vi "MagnetTop.vi"(8 "Queue to UI":T10, 11 "Module queue":T10) -> ()   [LabVIEW 2022 SP3, in "Magnet module.lvlib"]
doc: "Magnet module controls: power supply unit (PSU/SMS) and temperature monitor (TM/LSC218).\nPSU controls mainly: switch heater and ramping of current which runs throught coil.\nTM controls temperature of switch, coil and cryostat.\nMessage for magnet is a cluster that contains: {(enum) Command , (variant) Data}\nFor simplifieing of documentation, the Command is noted as a name of instruction, and Data is represented by a requered datatype (mostly cluster) name.\nCommands:\nInitialize(Magnet Config Constants) - Sugesstion: Load configuration constants from configuration file.\nSet field (Set field{B, R, cr}) - B-field[T], R-ramp[A/s], cr - custom ramp[bool].\nSwitch mode(mode) - to persistant, or to ramping.\nBlackout() - undone functionality of emergency deenergizing.\nUpdate() - Important! This triggers update of data from instruments. Shoud occure in regular intervals as priority message.\nResponses:\nMagnet initialized ();\nTM revision(temperature monitor revision);\nMagnet init error(error);\nSetting field(Set Field{B, R, cr});\nWarning(string);\nSwitching to(mode);\nUpdate error(error);\nTM update(TM sensors);\nPSU update(PSU data);\nMagnet status();"
uses:
  Magnet module.lvlib
  Messenger service/Data types/Mailbox address.ctl
  <instrlib>/SMS 120/Public/PSU Status.ctl
  ctl/Cryostat temperature sensors.ctl
  ctl/Overall status.ctl
  ctl/SetField data.ctl
  ctl/Magnet mode public.ctl
  ctl/Actual magnet state.ctl
  ctl/Magnet mode.ctl
  ctl/RampingOutput.ctl
  ctl/Magnet config constants.ctl
  Messenger service/Data types/Module name.ctl
  ctl/Magnet Orders.ctl
  ctl/MSG to magnet.ctl
  <instrlib>/SMS 120/Cryogenic Ltd SMSXXX.lvlib
  Messenger service/MessengerLib.lvlib
panel:
  out "Ended":bool=TRUE
  out "Magnet Constants":T1={"Switch resistant [K]"=5.0, "Switch superconducting [K]"=4.0, "First stage critical temperature [K]"=50.0, "Second stage critical temperature [K]"=5.0, "Inner magnet critical temperature [K]"=6.0, "Outer magnet critical temperature [K]"=5.0, "Field Constant [T/A]"=0.14911, "Maximum Current [A]"=107.3, "Maximum field [T]"=16.0, "Maximum source ramp [A/s]"=0.5, "Source precision [T]"=2e-05, "Ramp limits [A/s]"=[0.0506, 0.038, 0.0285, 0.0213, 0.0104], "Field limits [T]"=[3.0, 9.6, 13.3, 15.5, 16.0], "SMS"="", "LSC218"=""}
  out "Overall status":T2={"Desired"={"Field [T]"=0.0, "Ramp [T/s]"=0.0, "Custom Ramp?"=TRUE, "Mode"=enum."Persistant"}, "Actual"={"Mode"=enum."Persistant", "Ramping output"=enum."At Target", "Ready for change"=FALSE, "Switch heater"=FALSE, "Cooler Overheat"=FALSE, "Coil overheat"=FALSE, "Energized"=FALSE, "Output [T]"=0.0, "Field [T]"=0.0, "Ramp[T/s]"=0.0, "Switch\ntemperature [K]"=1.0, "Voltage [V]"=0.0, "Current direction"=FALSE}}
  out "Temperatures":T8[](array[typedef]) {"Time stamp" format="%<%H:%M:%S%2u\n%Y/%m/%d>T"}
  out "PSU Status Out":T9 {"Trip Current" format="%.3f"; "Trip Field" format="%.4f"; "Voltage" format="%.2f"; "Field Constant" format="%.6f"; "MID Setpoint (T)" format="%.4f"; "MID Setpoint (A)" format="%.3f"; "MAX Setpoint (T)" format="%.4f"; "MAX Setpoint (A)" format="%.3f"; "Heater Voltage" format="%.2f"; "V Limit (V)" format="%.2f"; "Ramp Rate (A/s)" format="%.3f"; "Output (A)" format="%.3f"; "Output (T)" format="%.4f"; "Persistent Current" format="%.3f"; "Persistent Field" format="%.4f"}
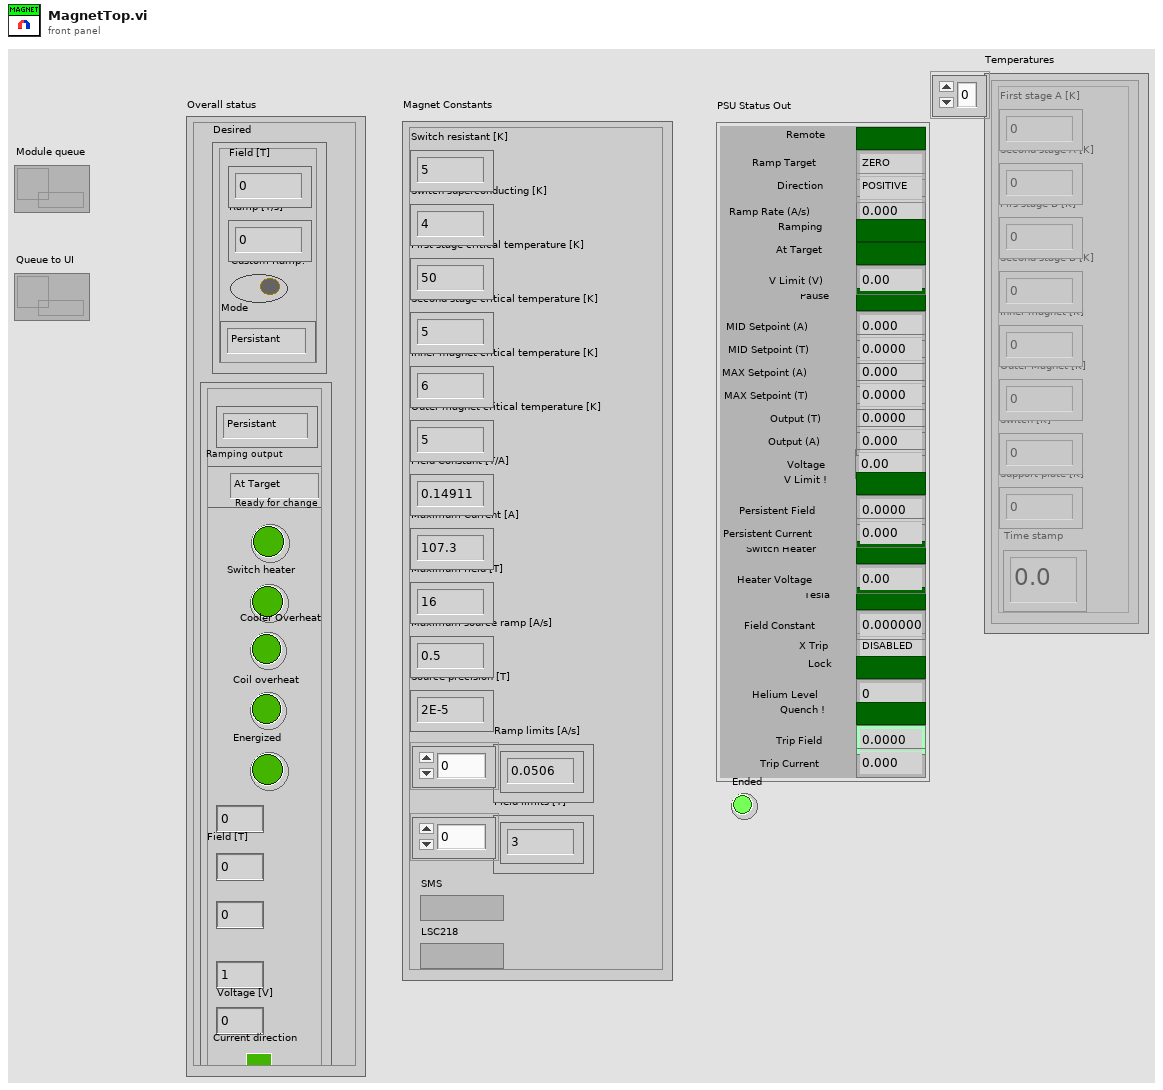
[diagram p1: front panel]
types:
  T1 = typedef "Magnet module.lvlib/Magnet config constants.ctl" = cluster{"Switch resistant [K]":dbl, "Switch superconducting [K]":dbl, "First stage critical temperature [K]":dbl, "Second stage critical temperature [K]":dbl, "Inner magnet critical temperature [K]":dbl, "Outer magnet critical temperature [K]":dbl, "Field Constant [T/A]":dbl, "Maximum Current [A]":dbl, "Maximum field [T]":dbl, "Maximum source ramp [A/s]":dbl, "Source precision [T]":dbl, "Ramp limits [A/s]":dbl[], "Field limits [T]":dbl[], "SMS":refnum<visa-resource-name>, "LSC218":refnum<visa-resource-name>}
  T2 = typedef "Magnet module.lvlib/Overall status.ctl" = cluster{"Desired":T3, "Actual":T5}
  T3 = typedef "Magnet module.lvlib/SetField data.ctl" = cluster{"Field [T]":dbl, "Ramp [T/s]":dbl, "Custom Ramp?":bool, "Mode":T4}
  T4 = typedef "Magnet module.lvlib/Magnet mode public.ctl" = enum16{"Persistant", "Ramping"}
  T5 = typedef "Magnet module.lvlib/Actual magnet state.ctl" = cluster{"Mode":T6, "Ramping output":T7, "Ready for change":bool, "Switch heater":bool, "Cooler Overheat":bool, "Coil overheat":bool, "Energized":bool, "Output [T]":dbl, "Field [T]":dbl, "Ramp[T/s]":dbl, "Switch\ntemperature [K]":dbl, "Voltage [V]":dbl, "Current direction":bool}
  T6 = typedef "Magnet module.lvlib/Magnet mode.ctl" = enum16{"Persistant", "Switching", "Ramping", "Quenched"}
  T7 = typedef "Magnet module.lvlib/RampingOutput.ctl" = enum16{"At Target", "Go up", "Go down"}
  T8 = typedef "Magnet module.lvlib/Cryostat temperature sensors.ctl" = cluster{"First stage A [K]":dbl, "Second stage A [K]":dbl, "Firs stage B [K]":dbl, "Second stage B [K]":dbl, "Inner magnet [K]":dbl, "Outer Magnet [K]":dbl, "Switch [K]":dbl, "Support plate [K]":dbl, "Time stamp":dbl}
  T9 = typedef "Cryogenic Ltd SMSXXX.lvlib/PSU Status.ctl" = cluster{"Ramp Target":enum16{"ZERO", "MID", "MAX"}, "Pause":bool, "Switch Heater":bool, "Persistent Field":dbl, "Persistent Current":dbl, "Tesla":bool, "Output (T)":dbl, "Output (A)":dbl, "X Trip":enum16{"DISABLED", "ENABLED", "ACTIVE"}, "Ramp Rate (A/s)":dbl, "V Limit (V)":dbl, "Heater Voltage":dbl, "MAX Setpoint (A)":dbl, "MAX Setpoint (T)":dbl, "MID Setpoint (A)":dbl, "MID Setpoint (T)":dbl, "Lock":bool, "Field Constant":dbl, "Remote":bool, "Direction":enum16{"POSITIVE", "NEGATIVE", "OPEN", "UNIPOLAR"}, "Helium Level":u16, "Quench !":bool, "Voltage":dbl, "V Limit !":bool, "Ramping":bool, "At Target":bool, "Trip Field":dbl, "Trip Current":dbl}
  T10 = typedef "MessengerLib.lvlib/Mailbox address.ctl" = refnum<queue>
  T11 = typedef "Magnet module.lvlib/MSG to magnet.ctl" = cluster{"Command":T12, "Data":variant}
  T12 = typedef "Magnet module.lvlib/Magnet Orders.ctl" = enum16{"Ignore", "Connect", "Update", "Switch mode", "Set field", "Stop ramping", "Equalize output", "Zero output", "Flip polarity", "Blackout", "Set timer", "Eval temperatures", "Disconnect"}
  T13 = typedef "Module name.ctl" = enum16{"Emty", "Magnet", "VTI", "Excitation", "Servo", "Acquisition", "Rotator", "Digitizer", "SMU2450", "Carousel", "Multimeter", "Tmp monitor", "Power monitor"}
  T14 = typedef "Magnet module.lvlib/TM Revision.ctl" = cluster{"Instr Serial Number":string, "Instr Driver Revision":string, "Instr Firmware Revision":string, "Instr Model Number":string}
  T15 = enum16{"POSITIVE", "NEGATIVE", "OPEN", "UNIPOLAR"}
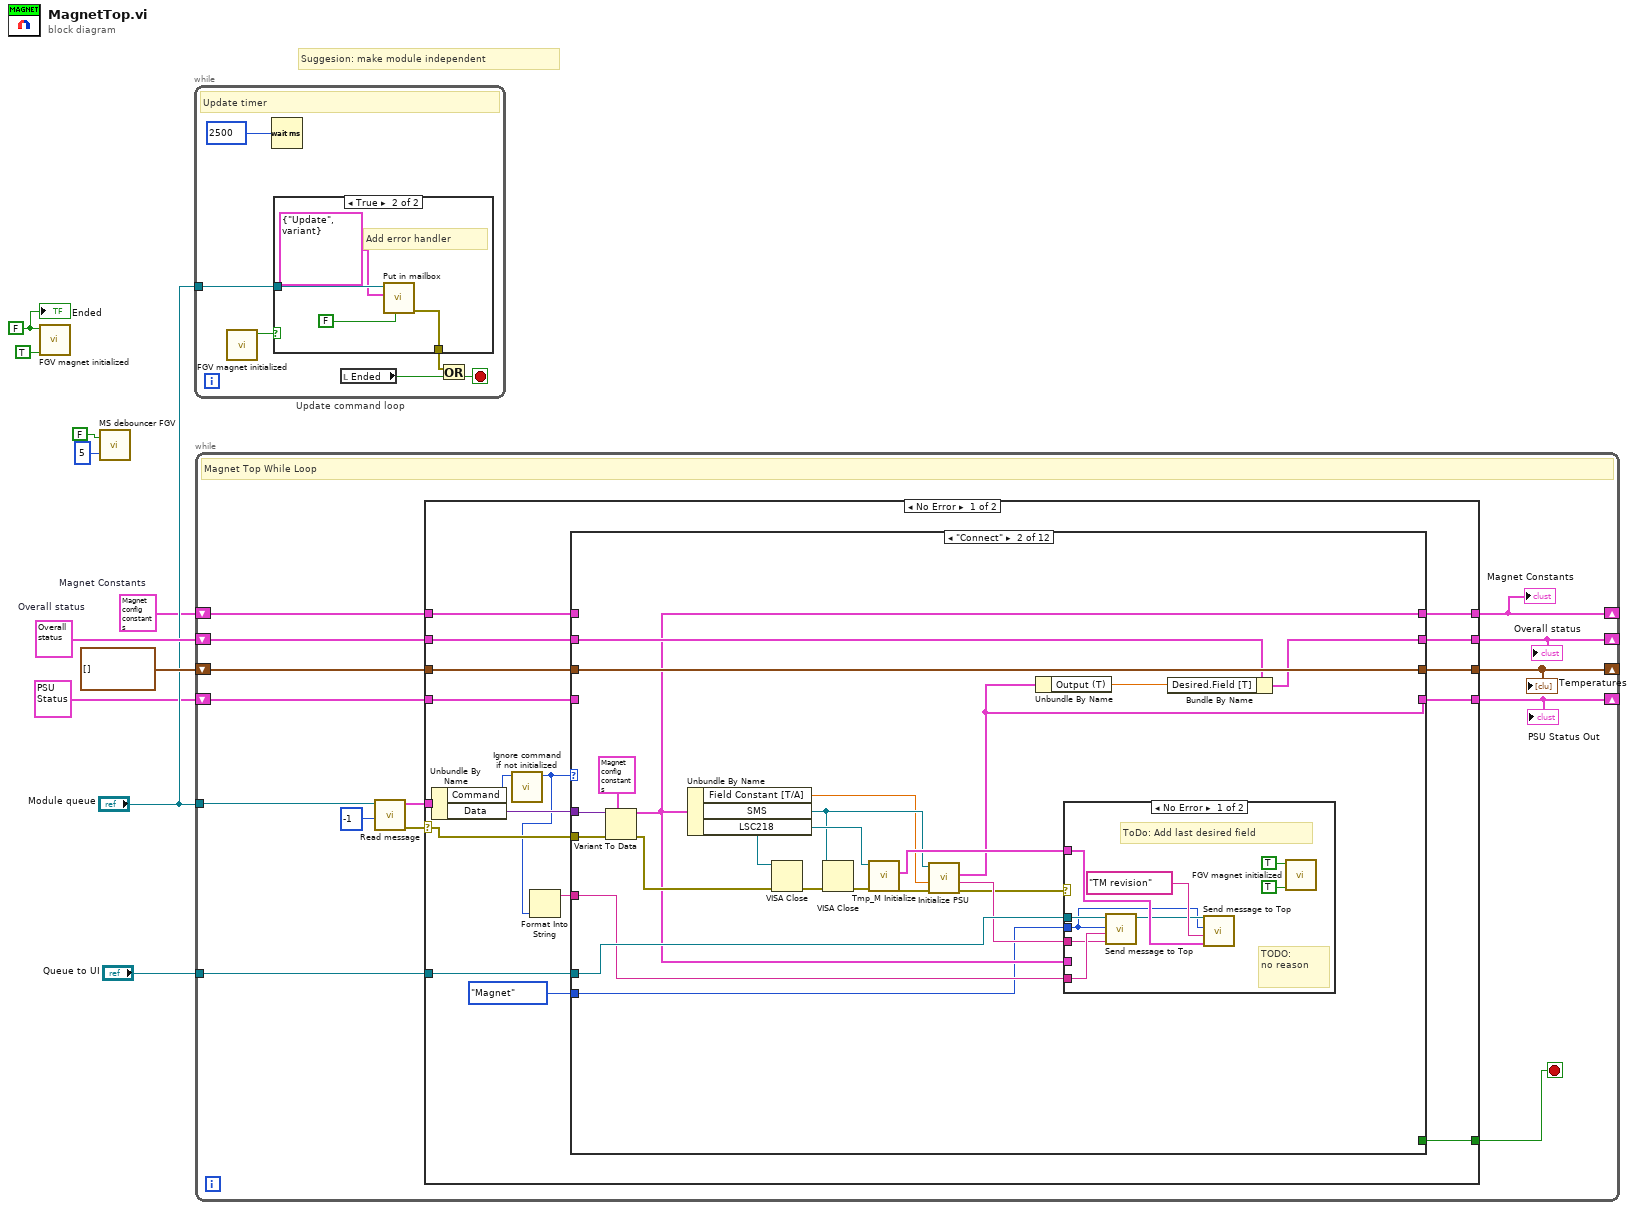
[diagram p0: block diagram]
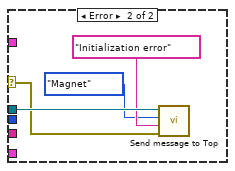
[diagram p4: hidden frame]
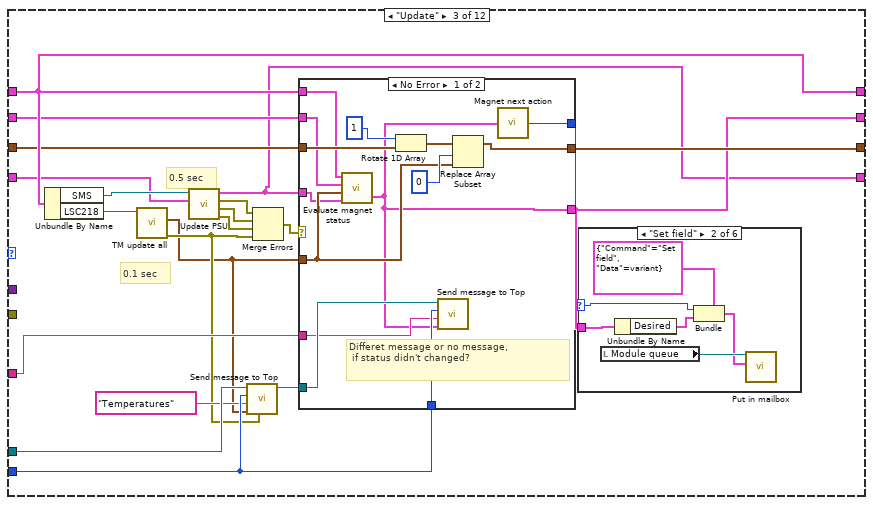
[diagram p5: hidden frame]
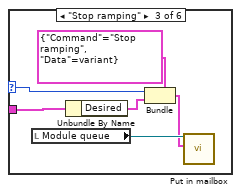
[diagram p7: hidden frame]
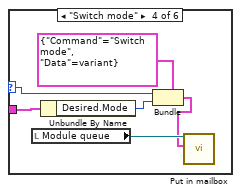
[diagram p8: hidden frame]
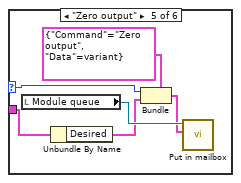
[diagram p9: hidden frame]
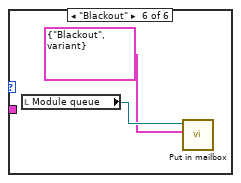
[diagram p10: hidden frame]
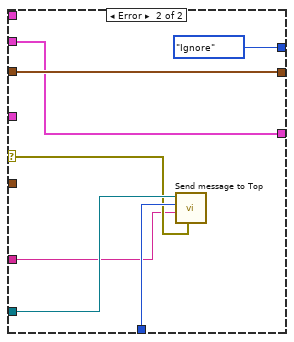
[diagram p11: hidden frame]
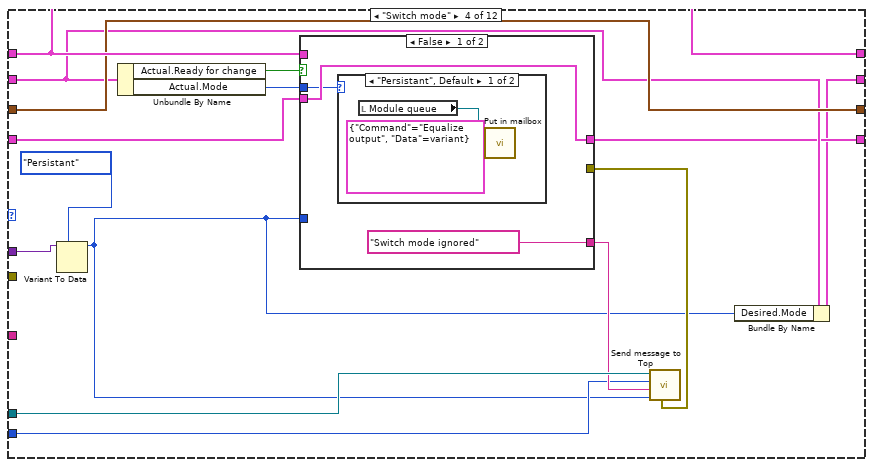
[diagram p12: hidden frame]
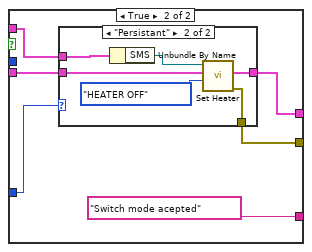
[diagram p14: hidden frame]
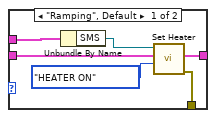
[diagram p15: hidden frame]
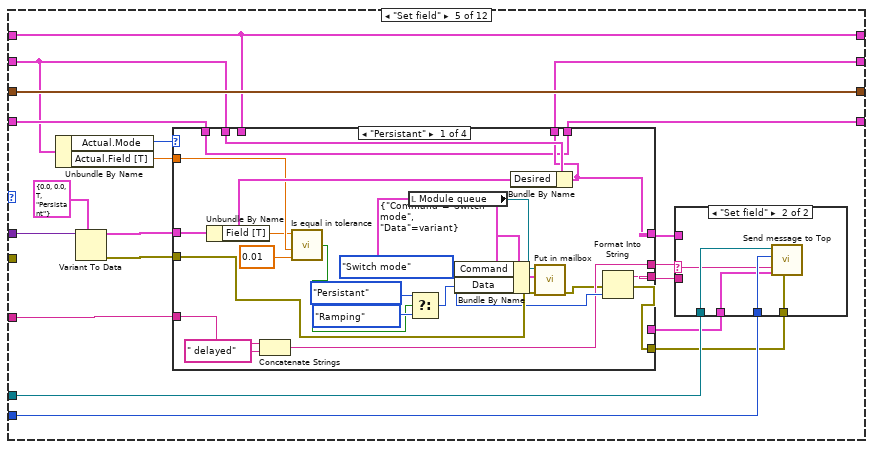
[diagram p16: hidden frame]
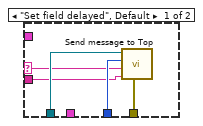
[diagram p17: hidden frame]
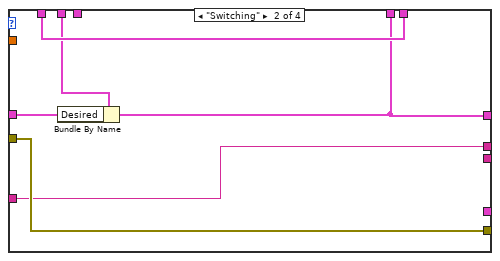
[diagram p18: hidden frame]
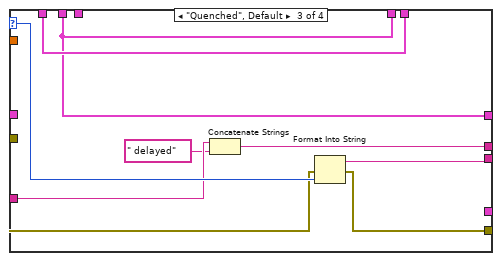
[diagram p19: hidden frame]
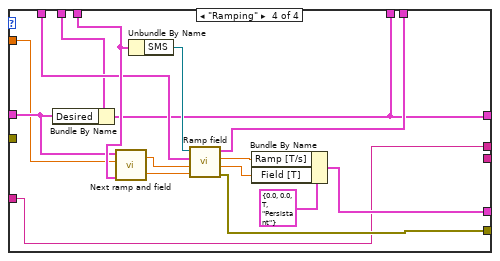
[diagram p20: hidden frame]
diagram:
  w1 = FALSE ("Initialized in")
  w2 = T1 {"Switch resistant [K]"=5.0, "Switch superconducting [K]"=4.0, "First stage critical temperature [K]"=50.0, "Second stage critical temperature [K]"=5.0, "Inner magnet critical temperature [K]"=6.0, "Outer magnet critical temperature [K]"=5.0, "Field Constant [T/A]"=0.14911, "Maximum Current [A]"=107.3, "Maximum field [T]"=16.0, "Maximum source ramp [A/s]"=0.5, "Source precision [T]"=2e-05, "Ramp limits [A/s]"=[0.0506, 0.038, 0.0285, 0.0213, 0.0104], "Field limits [T]"=[3.0, 9.6, 13.3, 15.5, 16.0], "SMS"="COM3", "LSC218"="COM1"}  # Magnet Constants
  w10 = T2 {"Desired"={"Field [T]"=0.0, "Ramp [T/s]"=0.0, "Custom Ramp?"=TRUE, "Mode"=enum."Persistant"}, "Actual"={"Mode"=enum."Persistant", "Ramping output"=enum."At Target", "Ready for change"=FALSE, "Switch heater"=FALSE, "Cooler Overheat"=FALSE, "Coil overheat"=FALSE, "Energized"=FALSE, "Output [T]"=0.0, "Field [T]"=0.0, "Ramp[T/s]"=0.0, "Switch\ntemperature [K]"=1.0, "Voltage [V]"=0.0, "Current direction"=FALSE}}  # Overall status
  # "Suggesion: make module independent"
  n1 = call "FGV magnet initialized.vi"("Write?(F)"=TRUE, "Initialized in"=w1) -> ()  [unwired: 9 in, 1 out]
  n2 = call "MS debouncer FGV.vi"("Iterations"=5, "At target?"=FALSE ("On target?")) -> ()  [unwired: 1 out]
  n3 = while "Update command loop" {
    tunnel: "Module queue" -> [w15]
    stop <- w12 stop-if-true
    # "Update timer"
    n4 = call "FGV magnet initialized.vi"() -> ("Initialized out"=w14:bool)  [unwired: 11 in]
    n5 = Wait (ms)(milliseconds to wait=u32 2500) -> ()  [unwired: 1 out]
    n6 = case shown="True" w14 {
      tunnel: w15 -> [_ w20]
      tunnel: [_ w17] -> w11
      frame False {
      }
      frame True {
        # "Add error handler"
        n7 = call "Put in mailbox.vi"("Priority? (F)"=FALSE ("Priority?"), "Message"=T11 {"Command"=enum."Update", "Data"=variant(enum16{"Ramping", "Perzistant"} enum."Ramping")} ("MSG to magnet"), "Queue in"=w20) -> ("error out"=w17:errorcluster)  [unwired: 6 in, 2 out]
      }
    }
    n8 = local read "Ended"() -> (w13:bool)
    n9 = Or(x=w11, y=w13) -> (x .or. y?=w12:bool)
  }
  n10 = while {
    tunnel: "Module queue" -> [w34]
    tunnel: "Queue to UI" -> [w33]
    shift-right: [w28] -> _
    shift-left: w10 -> [w29]
    shift-right: [w30] -> _
    shift-left: T8[] [] ("Temperatures") -> [w31]
    shift-right: [w27] -> _
    shift-left: T9 {"Ramp Target"=enum."ZERO", "Pause"=FALSE, "Switch Heater"=FALSE, "Persistent Field"=0.0, "Persistent Current"=0.0, "Tesla"=FALSE, "Output (T)"=0.0, "Output (A)"=0.0, "X Trip"=enum."DISABLED", "Ramp Rate (A/s)"=0.0, "V Limit (V)"=0.0, "Heater Voltage"=0.0, "MAX Setpoint (A)"=0.0, "MAX Setpoint (T)"=0.0, "MID Setpoint (A)"=0.0, "MID Setpoint (T)"=0.0, "Lock"=FALSE, "Field Constant"=0.0, "Remote"=FALSE, "Direction"=enum."POSITIVE", "Helium Level"=0, "Quench !"=FALSE, "Voltage"=0.0, "V Limit !"=FALSE, "Ramping"=FALSE, "At Target"=FALSE, "Trip Field"=0.0, "Trip Current"=0.0} ("PSU Status Out") -> [w26]
    shift-right: [w32] -> _
    shift-left: w2 -> [w25]
    stop <- w21 stop-if-true
    # "Magnet Top While Loop"
    n11 = call "Read message.vi"("timeout in ms (10)"=-1 ("timeout in ms (-1)"), "Module queue ref"=w34) -> ("error out"=w22:errorcluster, "MSG to magnet"=w23:T11)  [unwired: 8 in]
    n12 = case shown="No Error" w22 {
      selector: w22 -> [w40 _]
      tunnel: w33 -> [w51 _]
      tunnel: w23 -> [w44 _]
      tunnel: [w50 w473] -> w28
      tunnel: w29 -> [w49 w473]
      tunnel: w25 -> [w48 w474]
      tunnel: [w47 w474] -> w32
      tunnel: w31 -> [w46 w472]
      tunnel: [w45 w472] -> w30
      tunnel: [w43 w471] -> w27
      tunnel: w26 -> [w42 w471]
      tunnel: [w35 _] -> w21
      frame No Error {
        n13 = Unbundle By Name(w44) -> ("Command"=w36:T12, "Data"=w41:variant)
        n14 = call "Ignore command if not initialized.vi"("Command in"=w36) -> ("Command out"=w38:T12)  [unwired: 10 in]
        n15 = Format Into String(w38) -> (resulting string=w37:string)  [unwired: 3 in, 1 out]
        n16 = case shown="\"Connect\"" w38 {
          tunnel: w51 -> [_ w77 w100 w173 w212 w292 w322 w351 w383 _ w445 w459]
          tunnel: [w55 w71 w102 w160 w208 w289 w321 w353 w387 w432 w447 w461] -> w50
          tunnel: w49 -> [w55 w72 w106 w169 w207 w285 w321 w353 w387 w432 w447 w461]
          tunnel: w48 -> [w54 _ w107 w171 w199 w288 w326 w345 w378 w435 w446 w460]
          tunnel: [w54 w64 w107 w171 w199 w288 w326 w345 w378 w435 w446 w460] -> w47
          tunnel: w46 -> [w53 w76 w104 w170 w215 w293 w327 w354 w388 w434 w456 w470]
          tunnel: [w53 w76 w103 w170 w215 w293 w327 w354 w388 w434 w456 w470] -> w45
          tunnel: [w52 w70 w93 w167 w210 w286 w323 w348 w377 w433 w455 w469] -> w43
          tunnel: w42 -> [w52 _ w105 w168 w211 w287 w324 w349 w379 w433 w455 w469]
          tunnel: w41 -> [_ w68 _ w165 w213 _ _ _ w382 _ _ _]
          tunnel: w40 -> [_ w66 _ _ _ _ _ _ w381 _ _ _]
          tunnel: Module_name."Magnet" ("Module") -> [_ w62 w98 w164 w206 w291 _ w346 w385 _ _ _]
          tunnel: w37 -> [_ w63 w101 _ w200 w290 w318 w347 w384 _ w443 w457]
          tunnel: [_ _ _ _ _ _ _ _ _ _ w444 FALSE] -> w35
          frame "Ignore", Default {
          }
          frame "Connect" {
            n17 = Variant To Data(error in=w66, type=T1 {"Switch resistant [K]"=5.0, "Switch superconducting [K]"=4.0, "First stage critical temperature [K]"=50.0, "Second stage critical temperature [K]"=5.0, "Inner magnet critical temperature [K]"=6.0, "Outer magnet critical temperature [K]"=5.0, "Field Constant [T/A]"=0.14911, "Maximum Current [A]"=107.3, "Maximum field [T]"=16.0, "Maximum source ramp [A/s]"=0.5, "Source precision [T]"=2e-05, "Ramp limits [A/s]"=[0.0506, 0.038, 0.0285, 0.0213, 0.0104], "Field limits [T]"=[3.0, 9.6, 13.3, 15.5, 16.0], "SMS"="", "LSC218"=""} ("Magnet Config Constants"), Variant=w68) -> (data=w64:T1, error out=w65:errorcluster)
            n18 = Unbundle By Name(w64) -> ("Field Constant [T/A]"=w56:dbl, "SMS"=w59:refnum<visa-resource-name>, "LSC218"=w60:refnum<visa-resource-name>)
            n19 = VISA Close(VISA resource name=w60, error in (no error)=w65) -> (error out=w61:errorcluster)
            n20 = VISA Close(VISA resource name=w59, error in (no error)=w61) -> (error out=w57:errorcluster)
            n21 = call "Tmp_M Initialize.vi"("error in (no error)"=w57, "VISA Refnum in"=w60) -> ("error out"=w58:errorcluster, "TM Revision"=w75:T14)  [unwired: 7 in, 1 out]
            n22 = call "Initialize PSU.vi"("error in"=w58, "Field Constant"=w56, "PSU VISA name"=w59) -> ("error out"=w73:errorcluster, "Initial message"=w74:string, "initial PSU Status"=w70:T9)  [unwired: 6 in]
            n23 = Unbundle By Name(w70) -> ("Output (T)"=w69:dbl)
            n24 = case shown="No Error" w73 {
              selector: w73 -> [_ w89]
              tunnel: w77 -> [w82 w90]
              tunnel: w75 -> [w83 _]
              tunnel: w74 -> [w78 _]
              tunnel: w64 -> [_ _]
              tunnel: w63 -> [w80 _]
              tunnel: w62 -> [w79 _]
              frame No Error {
                # "TODO:\nno reason"
                # "ToDo: Add last desired field"
                n25 = call "Send message to Top.vi"("Data"=w78, "Response"=w80, "Module"=w79, "Mailbox address in"=w82) -> ("Mailbox address out"=w81:T10)  [unwired: 6 in, 1 out]
                n26 = call "Send message to Top.vi"("Data"=w83, "Response"="TM revision" ("Name"), "Module"=w79, "Mailbox address in"=w81) -> ()  [unwired: 6 in, 2 out]
                n27 = call "FGV magnet initialized.vi"("Write?(F)"=TRUE, "Initialized in"=TRUE) -> ()  [unwired: 9 in, 1 out]
              }
              frame Error {
                n28 = call "Send message to Top.vi"("Data"=w89, "Response"="Initialization error" ("Command"), "Module"=Module_name."Magnet", "Mailbox address in"=w90) -> ()  [unwired: 6 in, 2 out]
              }
            }
            n29 = Bundle By Name(cluster=w72, "Desired.Field [T]"=w69) -> (w71:T2)
          }
          frame "Update" {
            # "0.5 sec"
            # "0.1 sec"
            n30 = Unbundle By Name(w107) -> ("SMS"=w110:refnum<visa-resource-name>, "LSC218"=w111:refnum<visa-resource-name>)
            n31 = call "TM update all.vi"("VISA Refnum in"=w111) -> ("error out"=w96:errorcluster, "LSC218 sensors"=w95:T8)  [unwired: 8 in, 1 out]
            n32 = call "Update PSU.vi"("PSU Status In"=w105, "VISA Resource Name In"=w110) -> ("Output err"=w109:errorcluster, "Ramp state err"=w91:errorcluster, "Sign err"=w92:errorcluster, "PSU Status Out"=w93:T9)  [unwired: 2 in]
            n33 = call "Send message to Top.vi"("Error in (no error)"=w96, "Data"=w95, "Response"="Temperatures", "Module"=w98, "Mailbox address in"=w100) -> ("Mailbox address out"=w99:T10)  [unwired: 5 in, 1 out]
            n34 = Merge Errors(w92, w91, w109, w96) -> (w108:errorcluster)
            n35 = case shown="No Error" w108 {
              selector: w108 -> [_ w154]
              tunnel: w99 -> [w146 w157]
              tunnel: w95 -> [w143 _]
              tunnel: [w139 w156] -> w102
              tunnel: w104 -> [w149 w158]
              tunnel: [w147 w158] -> w103
              tunnel: w107 -> [w145 _]
              tunnel: w106 -> [w144 w156]
              tunnel: w98 -> [w142 w155]
              tunnel: w101 -> [w141 w153]
              tunnel: [w140 Magnet_Orders."Ignore" ("Command out")] -> w94
              tunnel: w93 -> [w138 _]
              frame No Error {
                # "Differet message or no message,\n if status didn't changed?"
                n36 = call "Evaluate magnet status.vi"("PSU Status in"=w138, "LSC218 sensors"=w143, "Overall status in"=w144, "Magnet Constants"=w145) -> ("Overall status out"=w139:T2)  [unwired: 1 in]
                n37 = Rotate 1D Array(1:w149, 2:1 ("n")) -> (0:w150:T8[])
                n38 = call "Send message to Top.vi"("Data"=w139, "Response"=w141, "Module"=w142, "Mailbox address in"=w146) -> ()  [unwired: 6 in, 2 out]
                n39 = Replace Array Subset(array=w150, new element=w143, index=0) -> (w147:T8[])
                n40 = call "Magnet next action.vi"("Overall status in"=w139) -> ("Command out"=w140:T12)  [unwired: 3 in, 1 out]
              }
              frame Error {
                n41 = call "Send message to Top.vi"("Error in (no error)"=w154, "Response"=w153, "Module"=w155, "Mailbox address in"=w157) -> ()  [unwired: 6 in, 2 out]
              }
            }
            n42 = case shown="\"Set field\"" w94 {
              selector: w94 -> [_ w112 w118 w124 w130 _]
              tunnel: w102 -> [_ w114 w120 w126 w132 _]
              frame "Update", Default {
              }
              frame "Set field" {
                n43 = local read "Module queue"() -> (w117:T10)
                n44 = Unbundle By Name(w114) -> ("Desired"=w115:T3)
                n45 = Bundle(cluster=T11 {"Command"=enum."Set field", "Data"=variant} ("MSG to magnet"), "Command"=w112, "Data"=w115) -> (w113:T11)
                n46 = call "Put in mailbox.vi"("Message"=w113, "Queue in"=w117) -> ()  [unwired: 7 in, 3 out]
              }
              frame "Stop ramping" {
                n47 = local read "Module queue"() -> (w123:T10)
                n48 = Unbundle By Name(w120) -> ("Desired"=w121:T3)
                n49 = Bundle(cluster=T11 {"Command"=enum."Stop ramping", "Data"=variant} ("MSG to magnet"), "Command"=w118, "Data"=w121) -> (w119:T11)
                n50 = call "Put in mailbox.vi"("Message"=w119, "Queue in"=w123) -> ()  [unwired: 7 in, 3 out]
              }
              frame "Switch mode" {
                n51 = local read "Module queue"() -> (w129:T10)
                n52 = Unbundle By Name(w126) -> ("Desired.Mode"=w127:T4)
                n53 = Bundle(cluster=T11 {"Command"=enum."Switch mode", "Data"=variant} ("MSG to magnet"), "Command"=w124, "Data"=w127) -> (w125:T11)
                n54 = call "Put in mailbox.vi"("Message"=w125, "Queue in"=w129) -> ()  [unwired: 7 in, 3 out]
              }
              frame "Zero output" {
                n55 = local read "Module queue"() -> (w135:T10)
                n56 = Unbundle By Name(w132) -> ("Desired"=w133:T3)
                n57 = Bundle(cluster=T11 {"Command"=enum."Zero output", "Data"=variant} ("MSG to magnet"), "Command"=w130, "Data"=w133) -> (w131:T11)
                n58 = call "Put in mailbox.vi"("Message"=w131, "Queue in"=w135) -> ()  [unwired: 7 in, 3 out]
              }
              frame "Blackout" {
                n59 = local read "Module queue"() -> (w137:T10)
                n60 = call "Put in mailbox.vi"("Message"=T11 {"Command"=enum."Blackout", "Data"=variant} ("MSG to magnet"), "Queue in"=w137) -> ()  [unwired: 7 in, 3 out]
              }
            }
          }
          frame "Switch mode" {
            n61 = Variant To Data(type=Magnet_mode_public."Persistant" ("Desired.Mode"), Variant=w165) -> (data=w159:T4)  [unwired: 1 in, 1 out]
            n62 = Unbundle By Name(w169) -> ("Actual.Ready for change"=w172:bool, "Actual.Mode"=w163:T6)
            n63 = case shown="False" w172 {
              tunnel: w159 -> [_ w183]
              tunnel: w171 -> [_ w184]
              tunnel: w168 -> [w176 w182]
              tunnel: [w176 w181] -> w167
              tunnel: ["Switch mode ignored" ("Name") "Switch mode acepted" ("Name")] -> w166
              tunnel: w163 -> [w174 _]
              tunnel: [_ w179] -> w162
              frame False {
                n64 = case shown="\"Persistant\", Default" w174 {
                  frame "Persistant", Default {
                    n65 = local read "Module queue"() -> (w177:T10)
                    n66 = call "Put in mailbox.vi"("Message"=T11 {"Command"=enum."Equalize output", "Data"=variant(enum16{"Ramping", "Perzistant"} enum."Ramping")} ("MSG to magnet"), "Queue in"=w177) -> ()  [unwired: 7 in, 3 out]
                  }
                  frame "Ramping" {
                  }
                }
              }
              frame True {
                n67 = case shown="\"Persistant\"" w183 {
                  tunnel: w184 -> [w188 w194]
                  tunnel: w182 -> [w187 w193]
                  tunnel: [w186 w192] -> w181
                  tunnel: [w185 w191] -> w179
                  frame "Ramping", Default {
                    n68 = Unbundle By Name(w188) -> ("SMS"=w190:refnum<visa-resource-name>)
                    n69 = call <instrlib>:"Set Heater.vi"("Heater (On/Off)"=enum16{"HEATER OFF", "HEATER ON"}."HEATER ON", "PSU Status In"=w187, "VISA Resource Name In"=w190) -> ("Error out"=w185:errorcluster, "PSU Status Out"=w186:T9)  [unwired: 5 in, 2 out]
                  }
                  frame "Persistant" {
                    n70 = Unbundle By Name(w194) -> ("SMS"=w196:refnum<visa-resource-name>)
                    n71 = call <instrlib>:"Set Heater.vi"("Heater (On/Off)"=enum16{"HEATER OFF", "HEATER ON"}."HEATER OFF", "PSU Status In"=w193, "VISA Resource Name In"=w196) -> ("Error out"=w191:errorcluster, "PSU Status Out"=w192:T9)  [unwired: 5 in, 2 out]
                  }
                }
              }
            }
            n72 = call "Send message to Top.vi"("Error in (no error)"=w162, "Data"=w159, "Response"=w166, "Module"=w164, "Mailbox address in"=w173) -> ()  [unwired: 5 in, 2 out]
            n73 = Bundle By Name(cluster=w169, "Desired.Mode"=w159) -> (w160:T2)
          }
          frame "Set field" {
            n74 = Unbundle By Name(w207) -> ("Actual.Mode"=w216:T6, "Actual.Field [T]"=w198:dbl)
            n75 = Variant To Data(type=T3 {"Field [T]"=0.0, "Ramp [T/s]"=0.0, "Custom Ramp?"=TRUE, "Mode"=enum."Persistant"} ("Set Field"), Variant=w213) -> (data=w209:T3, error out=w205:errorcluster)  [unwired: 1 in]
            n76 = case shown="\"Persistant\"" w216 {
              selector: w216 -> [_ _ w259 _]
              tunnel: w207 -> [w248 w252 w262 w269]
              tunnel: w199 -> [_ _ _ w279]
              tunnel: w211 -> [w246 w254 w263 w278]
              tunnel: [w246 w254 w263 w277] -> w210
              tunnel: w209 -> [w234 w251 _ w276]
              tunnel: [w247 w250 w262 w267] -> w208
              tunnel: w205 -> [w242 w253 w258 _]
              tunnel: [w247 w250 w262 w267] -> w204
              tunnel: [w238 w249 w261 w265] -> w203
              tunnel: [w235 w253 w257 w268] -> w202
              tunnel: [_ _ _ w266] -> w201
              tunnel: w200 -> [w240 w249 w256 w265]
              tunnel: w198 -> [w233 _ _ w264]
              tunnel: [w237 _ w260 _] -> w197
              frame "Persistant" {
                w239 = Magnet_Orders."Switch mode" ("Order")
                n77 = Unbundle By Name(w234) -> ("Field [T]"=w232:dbl)
                n78 = Concatenate Strings(w240, " delayed" ("string")) -> (w238:string)
                n79 = call "Is equal in tolerance.vi"("Absolut tolerance"=0.01, "Reference value"=w233, "Input value"=w232) -> ("Is in range"=w228:bool)  [unwired: 1 in]
                n80 = local read "Module queue"() -> (w243:T10)
                n81 = Select(t=Magnet_mode_public."Persistant" ("Operation mode"), s=w228, f=Magnet_mode_public."Ramping" ("Operation mode")) -> (s? t:f=w227:T4)
                n82 = Bundle By Name(cluster=T11 {"Command"=enum."Switch mode", "Data"=variant(enum16{"Ramping", "Perzistant"} enum."Ramping")} ("MSG to magnet"), "Command"=w239, "Data"=w227) -> (w245:T11)
                n83 = Bundle By Name(cluster=w248, "Desired"=w234) -> (w247:T2)
                n84 = call "Put in mailbox.vi"("error in (no error)"=w242, "Message"=w245, "Queue in"=w243) -> ("error out"=w236:errorcluster)  [unwired: 6 in, 2 out]
                n85 = Format Into String(error in=w236, w239) -> (resulting string=w237:string, error out=w235:errorcluster)  [unwired: 2 in]
              }
              frame "Switching" {
                n86 = Bundle By Name(cluster=w252, "Desired"=w251) -> (w250:T2)
              }
              frame "Quenched", Default {
                n87 = Concatenate Strings(w256, " delayed" ("string")) -> (w261:string)
                n88 = Format Into String(error in=w258, w259) -> (resulting string=w260:string, error out=w257:errorcluster)  [unwired: 2 in]
              }
              frame "Ramping" {
                n89 = Bundle By Name(cluster=w269, "Desired"=w276) -> (w267:T2)
                n90 = call "Next ramp and field.vi"("Magnet Constants in"=w279, "Actual field [T]"=w264, "Desired"=w276) -> ("Ramp to set [A/s]"=w273:dbl, "Field to set [T]"=w274:dbl)  [unwired: 1 in]
                n91 = Unbundle By Name(w279) -> ("SMS"=w275:refnum<visa-resource-name>)
                n92 = call "Ramp field.vi"("Ramp to set [A/s]"=w273, "Field to set [T]"=w274, "PSU Status In"=w278, "VISA Refnum in"=w275) -> ("error out"=w268:errorcluster, "Desired field (T)"=w271:dbl, "Ramp Rate (T/s)"=w272:dbl, "PSU Status Out"=w277:T9)  [unwired: 4 in]
                n93 = Bundle By Name(cluster=T3 {"Field [T]"=0.0, "Ramp [T/s]"=0.0, "Custom Ramp?"=TRUE, "Mode"=enum."Persistant"} ("Desired"), "Ramp [T/s]"=w272, "Field [T]"=w271) -> (w266:T3)
              }
            }
            n94 = case shown="\"Set field\"" w203 {
              selector: w203 -> [w219 w223]
              tunnel: w212 -> [w221 w226]
              tunnel: w206 -> [w220 w225]
              tunnel: w202 -> [w218 w224]
              tunnel: w204 -> [_ _]
              tunnel: w201 -> [_ w222]
              tunnel: w197 -> [w217 _]
              frame "Set field delayed", Default {
                n95 = call "Send message to Top.vi"("Error in (no error)"=w218, "Data"=w217, "Response"=w219, "Module"=w220, "Mailbox address in"=w221) -> ()  [unwired: 5 in, 2 out]
              }
              frame "Set field" {
                n96 = call "Send message to Top.vi"("Error in (no error)"=w224, "Data"=w222, "Response"=w223, "Module"=w225, "Mailbox address in"=w226) -> ()  [unwired: 5 in, 2 out]
              }
            }
          }
          frame "Stop ramping" {
            n97 = Unbundle By Name(w285) -> ("Desired.Field [T]"=w284:dbl)
            n98 = call "Is equal in tolerance.vi"("Absolut tolerance"=0.001, "Reference value"=0.0, "Input value"=w284) -> ("Is in range"=w281:bool)  [unwired: 1 in]
            n99 = case shown="False" w281 {
              tunnel: [w314 w316] -> w289
              tunnel: w288 -> [w313 _]
              tunnel: w287 -> [w306 w317]
              tunnel: [w300 w317] -> w286
              tunnel: w285 -> [w298 w316]
              tunnel: [w296 "Field is discharging"] -> w280
              frame False {
                n100 = Unbundle By Name(w313) -> ("SMS"=w309:refnum<visa-resource-name>)
                n101 = call <instrlib>:"Set Pause.vi"("Pause (On/Off)"=enum16{"PAUSE OFF", "PAUSE ON"}."PAUSE ON", "PSU Status In"=w306, "VISA Resource Name IN"=w309) -> ("Error out"=w304:errorcluster, "PSU Status Out"=w305:T9, "VISA Resource Name Out"=w308:refnum<visa-resource-name>)  [unwired: 5 in, 1 out]
                n102 = call <instrlib>:"Get Output.vi"("Error in (no error)"=w304, "PSU Status In"=w305, "VISA Resource Name In"=w308) -> ("Error out"=w311:errorcluster, "PSU Status Out"=w312:T9, "VISA Resource Name Out"=w310:refnum<visa-resource-name>, "Output (T)"=w294:dbl)  [unwired: 3 in, 2 out]
                n103 = call <instrlib>:"Set MID.vi"("Error in (no error)"=w311, "MID (T or A)"=w294, "PSU Status In"=w312, "VISA Resource Name In"=w310) -> ("Error out"=w303:errorcluster, "PSU Status Out"=w301:T9, "VISA Resource Name Out"=w302:refnum<visa-resource-name>)  [unwired: 4 in, 1 out]
                n104 = Bundle By Name(cluster=w298, "Desired.Field [T]"=w294) -> (w314:T2)
                n105 = Format Into String(format string="%f T", initial string="Field stopped at ", w294) -> (resulting string=w296:string)  [unwired: 1 in, 1 out]
                n106 = call <instrlib>:"Set Pause.vi"("Error in (no error)"=w303, "Pause (On/Off)"=enum16{"PAUSE OFF", "PAUSE ON"}."PAUSE OFF", "PSU Status In"=w301, "VISA Resource Name IN"=w302) -> ("PSU Status Out"=w300:T9)  [unwired: 4 in, 3 out]
              }
              frame True {
              }
            }
            n107 = call "Send message to Top.vi"("Data"=w280, "Response"=w290, "Module"=w291, "Mailbox address in"=w292) -> ()  [unwired: 6 in, 2 out]
          }
          frame "Equalize output" {
            n108 = Unbundle By Name(w326) -> ("SMS"=w325:refnum<visa-resource-name>)
            n109 = Unbundle By Name(w321) -> ("Actual.Field [T]"=w319:dbl, "Actual.Mode"=w320:T6)
            n110 = case shown="\"Persistant\"" w320 {
              tunnel: w325 -> [w338 _]
              tunnel: w319 -> [w331 _]
              tunnel: w324 -> [w337 w343]
              tunnel: [w336 w343] -> w323
              tunnel: w322 -> [w334 w342]
              tunnel: w318 -> [w328 w340]
              frame "Persistant" {
                n111 = call "Ramp field.vi"("Ramp to set [A/s]"=0.5, "Field to set [T]"=w331, "PSU Status In"=w337, "VISA Refnum in"=w338) -> ("Ramp Rate (T/s)"=w329:dbl, "PSU Status Out"=w336:T9)  [unwired: 4 in, 2 out]
                n112 = Bundle By Name(cluster=T3 {"Field [T]"=0.0, "Ramp [T/s]"=0.0, "Custom Ramp?"=TRUE, "Mode"=enum."Persistant"} ("Desired"), "Field [T]"=w331, "Ramp [T/s]"=w329) -> (w330:T3)
                n113 = call "Send message to Top.vi"("Data"=w330, "Response"=w328, "Module"=Module_name."Magnet", "Mailbox address in"=w334) -> ()  [unwired: 6 in, 2 out]
              }
              frame "Ramping", Default {
                n114 = call "Send message to Top.vi"("Data"=T3 {"Field [T]"=0.0, "Ramp [T/s]"=0.0, "Custom Ramp?"=TRUE, "Mode"=enum."Ramping"} ("Desired"), "Response"=w340, "Module"=Module_name."Magnet", "Mailbox address in"=w342) -> ()  [unwired: 6 in, 2 out]
              }
            }
          }
          frame "Zero output" {
            n115 = Unbundle By Name(w353) -> ("Actual.Field [T]"=w344:dbl, "Actual.Mode"=w352:T6)
            n116 = Unbundle By Name(w345) -> ("SMS"=w350:refnum<visa-resource-name>)
            n117 = case shown="\"Persistant\"" w352 {
              tunnel: w351 -> [w363 w375]
              tunnel: w350 -> [w362 w364]
              tunnel: w349 -> [w361 w369]
              tunnel: [w360 w368] -> w348
              tunnel: w347 -> [w357 w373]
              tunnel: w346 -> [w355 w372]
              tunnel: w345 -> [_ w366]
              tunnel: w344 -> [_ w365]
              frame "Persistant" {
                n118 = call "Ramp field.vi"("Ramp to set [A/s]"=0.5, "Field to set [T]"=0.0, "PSU Status In"=w361, "VISA Refnum in"=w362) -> ("PSU Status Out"=w360:T9)  [unwired: 4 in, 3 out]
                n119 = call "Send message to Top.vi"("Data"=TRUE, "Response"=w357, "Module"=w355, "Mailbox address in"=w363) -> ()  [unwired: 6 in, 2 out]
              }
              frame "Ramping", Default {
                n120 = call "Next ramp and field.vi"("Magnet Constants in"=w366, "Actual field [T]"=w365, "Desired"=T3 {"Field [T]"=0.0, "Ramp [T/s]"=0.0, "Custom Ramp?"=FALSE, "Mode"=enum."Ramping"}) -> ("Ramp to set [A/s]"=w370:dbl, "Field to set [T]"=w371:dbl)  [unwired: 1 in]
                n121 = call "Ramp field.vi"("Ramp to set [A/s]"=w370, "Field to set [T]"=w371, "PSU Status In"=w369, "VISA Refnum in"=w364) -> ("PSU Status Out"=w368:T9)  [unwired: 4 in, 3 out]
                n122 = call "Send message to Top.vi"("Data"=FALSE, "Response"=w373, "Module"=w372, "Mailbox address in"=w375) -> ()  [unwired: 6 in, 2 out]
              }
            }
          }
          frame "Flip polarity" {
            n123 = Unbundle By Name(w387) -> ("Actual.Mode"=w386:T6)
            n124 = Variant To Data(error in=w381, type=TRUE, Variant=w382) -> (data=w376:bool)  [unwired: 1 out]
            n125 = case shown="\"Ramping\"" w386 {
              tunnel: w385 -> [w392 w406]
              tunnel: w384 -> [w391 w405]
              tunnel: w383 -> [w390 w404]
              tunnel: w379 -> [w393 w400]
              tunnel: [w393 w403] -> w377
              tunnel: w378 -> [_ w402]
              tunnel: w376 -> [_ w399]
              frame "Persistant", Default {
                n126 = call "Send message to Top.vi"("Data"="Cannot flip polarity", "Response"=w391, "Module"=w392, "Mailbox address in"=w390) -> ()  [unwired: 6 in, 2 out]
              }
              frame "Ramping" {
                n127 = Unbundle By Name(w400) -> ("Direction"=w394:T15)
                n128 = case shown="\"OPEN\"" w394 {
                  tunnel: w399 -> [w421 w424 _ _]
                  tunnel: [w420 w424 _ _] -> w398
                  tunnel: [enum16{"NEGATIVE", "POSITIVE"}."NEGATIVE" ("Current Direction") enum16{"NEGATIVE", "POSITIVE"}."POSITIVE" ("Current Direction") enum16{"NEGATIVE", "POSITIVE"}."POSITIVE" ("Current Direction") enum16{"NEGATIVE", "POSITIVE"}."POSITIVE" ("Current Direction")] -> w397
                  frame "POSITIVE", Default {
                    n129 = Not(x=w421) -> (.not. x?=w420:bool)
                  }
                  frame "NEGATIVE" {
                  }
                  frame "OPEN" {
                  }
                  frame "UNIPOLAR" {
                  }
                }
                n130 = Unbundle By Name(w402) -> ("SMS"=w401:refnum<visa-resource-name>)
                n131 = case shown="True" w398 {
                  tunnel: [w414 w417] -> w403
                  tunnel: w401 -> [w413 _]
                  tunnel: w400 -> [w412 w417]
                  tunnel: w397 -> [w410 _]
                  tunnel: [w409 w419] -> w396
                  tunnel: [w408 w418] -> w395
                  tunnel: w394 -> [_ w416]
                  frame True {
                    n132 = call <instrlib>:"Set Current Direction.vi"("Current Direction"=w410, "PSU Status In"=w412, "VISA Resource Name In"=w413) -> ("Error out"=w411:errorcluster, "PSU Status Out"=w414:T9)  [unwired: 5 in, 2 out]
                    n133 = Format Into String(format string="Set polarity: %s", error in=w411, w410) -> (resulting string=w409:string, error out=w408:errorcluster)  [unwired: 1 in]
                  }
                  frame False {
                    n134 = Format Into String(format string="Polarity is %s", w416) -> (resulting string=w419:string, error out=w418:errorcluster)  [unwired: 2 in]
                  }
                }
                n135 = call "Send message to Top.vi"("Error in (no error)"=w395, "Data"=w396, "Response"=w405, "Module"=w406, "Mailbox address in"=w404) -> ()  [unwired: 5 in, 2 out]
              }
            }
          }
          frame "Blackout" {
            n136 = Unbundle By Name(w432) -> ("Actual.Mode"=w430:T6, "Actual.Energized"=w431:bool, "Desired.Field [T]"=w427:dbl)
            n137 = Not Equal To 0?(x=w427) -> (x != 0?=w428:bool)
            n138 = And(x=w431, y=w428) -> (x .and. y?=w429:bool)
            n139 = case shown="True" w429 {
              tunnel: w430 -> [_ w436]
              frame False {
              }
              frame True {
                n140 = case shown="\"Persistant\", Default" w436 {
                  frame "Persistant", Default {
                    n141 = local read "Module queue"() -> (w442:T10)
                    n142 = Bundle(cluster=T11 {"Command"=enum."Set field", "Data"=variant} ("MSG to magnet"), "Command"=Magnet_Orders."Set field" ("Order"), "Data"=T3 {"Field [T]"=0.0, "Ramp [T/s]"=1.0, "Custom Ramp?"=FALSE, "Mode"=enum."Ramping"} ("Set Field")) -> (w441:T11)
                    n143 = call "Put in mailbox.vi"("Priority? (F)"=TRUE, "Message"=w441, "Queue in"=w442) -> ()  [unwired: 6 in, 3 out]
                  }
                  frame "Quenched" {
                  }
                }
              }
            }
          }
          frame "Eval temperatures" {
            w444 = TRUE
            n144 = Unbundle By Name(w446) -> ("LSC218"=w450:refnum<visa-resource-name>, "SMS"=w454:refnum<visa-resource-name>)
            n145 = VISA Close(VISA resource name=w454) -> (error out=w449:errorcluster)  [unwired: 1 in]
            n146 = VISA Close(VISA resource name=w450, error in (no error)=w449) -> (error out=w448:errorcluster)
            n147 = call "Send message to Top.vi"("Data"=w448, "Response"=w443, "Module"=Module_name."Magnet", "Mailbox address in"=w445) -> ()  [unwired: 6 in, 2 out]
            n148 = call "FGV magnet initialized.vi"("Write?(F)"=TRUE, "Initialized in"=FALSE) -> ()  [unwired: 9 in, 1 out]
            n149 = local write "Ended"(w444) -> ()
          }
          frame "Disconnect" {
            n150 = Unbundle By Name(w460) -> ("LSC218"=w464:refnum<visa-resource-name>, "SMS"=w468:refnum<visa-resource-name>)
            n151 = VISA Close(VISA resource name=w468) -> (error out=w463:errorcluster)  [unwired: 1 in]
            n152 = VISA Close(VISA resource name=w464, error in (no error)=w463) -> (error out=w462:errorcluster)
            n153 = call "Send message to Top.vi"("Data"=w462, "Response"=w457, "Module"=Module_name."Magnet", "Mailbox address in"=w459) -> ()  [unwired: 6 in, 2 out]
            n154 = call "FGV magnet initialized.vi"("Write?(F)"=TRUE, "Initialized in"=FALSE) -> ()  [unwired: 9 in, 1 out]
          }
        }
      }
      frame Error {
      }
    }
    "PSU Status Out" <- w27
    "Temperatures" <- w30
    "Overall status" <- w28
    "Magnet Constants" <- w32
  }
  "Ended" <- w1
